vi "Main.vi"   [LabVIEW 2024]
doc: "Main VI"
uses:
  controls/GlobalData.vi
  support/Message Queue/Message Queue.lvlib
types:
  T1 = typedef "Message Queue.lvlib/All Message Queues.ctl" = cluster{"Processing":refnum<queue>, "Data Log":refnum<queue>, "RS232 Sim":refnum<queue>}
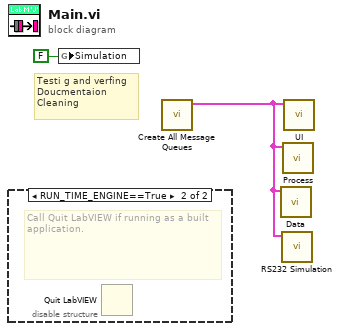
[diagram p0: block diagram]
diagram:
  # "Testi g and verfing \nDoucmentaion\nCleaning"
  n1 = disable-structure shown="RUN_TIME_ENGINE==True" {
    frame condition #0 (active) {
    }
    frame condition #1 {
      # "Call Quit LabVIEW if running as a built application."
      n2 = Quit LabVIEW() -> ()  [unwired: 1 in]
    }
  }
  n3 = global write "GlobalData.vi" "Simulation"(FALSE ("Simulation")) -> ()
  n4 = call "Create All Message Queues.vi"() -> ("Message Queues out"=w1:T1)  [unwired: 10 in, 1 out]
  n5 = call "Data.vi"("Message Queues out"=w1) -> ()  [unwired: 11 in]
  n6 = call "RS232 Simulation.vi"("Message Queues out"=w1) -> ()  [unwired: 11 in]
  n7 = call "Process.vi"("Message Queues out"=w1) -> ()  [unwired: 11 in]
  n8 = call "UI.vi"("Message Queues out"=w1) -> ()  [unwired: 11 in]
